vi "geve-init.vi"(8 "error in (no error)":errorcluster) -> (0 "error out":errorcluster, 3 "Runtime Data":T1)   [LabVIEW 2018]
doc: "perfoms action :\ninit com references,\nenqueue message append init message to log\nget configuration from cfg file, enqueue message to log info and to update data in main cluster\nenqueue message to open serial com."
uses:
  geve-runtime_data_cluster.ctl
  geve-monitoring_data_cluster.ctl
  geve-serial_config_cluster.ctl
  geve-com_ref_cluster.ctl
  geve-message_cluster.ctl
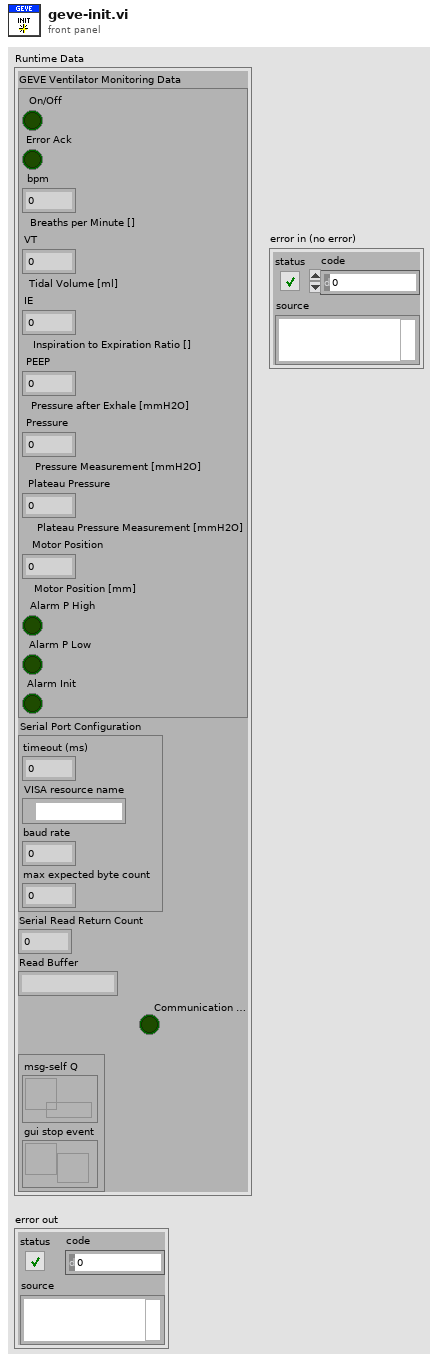
[diagram p1: front panel]
types:
  T1 = typedef "geve-runtime_data_cluster.ctl" = cluster{"GEVE Ventilator Monitoring Data":T2, "Serial Port Configuration":T3, "Serial Read Return Count":u32, "Read Buffer":string, "Communication Timeout?":bool, "com-refs":T4}
  T2 = typedef "geve-monitoring_data_cluster.ctl" = cluster{"On/Off":bool, "Error Ack":bool, "bpm":dbl, "VT":dbl, "IE":dbl, "PEEP":dbl, "Pressure":dbl, "Plateau Pressure":dbl, "Motor Position":dbl, "Alarm P High":bool, "Alarm P Low":bool, "Alarm Init":bool}
  T3 = typedef "geve-serial_config_cluster.ctl" = cluster{"timeout (ms)":u32, "VISA resource name":refnum<visa-resource-name>, "baud rate":u32, "max expected byte count":u32}
  T4 = typedef "geve-com_ref_cluster.ctl" = cluster{"msg-self Q":refnum<queue>, "gui stop event":refnum<user-event>}
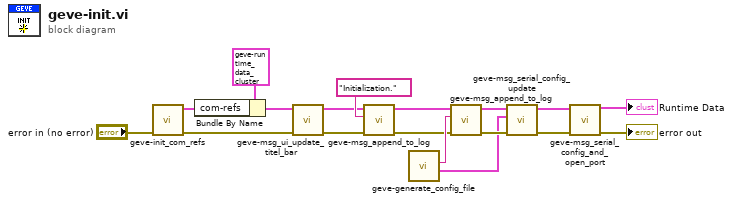
[diagram p0: block diagram]
diagram:
  n1 = call "geve-init_com_refs.vi"("error in (no error)"="error in (no error)") -> ("error out"=w10:errorcluster, "com-refs"=w8:T4)  [unwired: 9 in]
  n2 = Bundle By Name(cluster=T1 {"GEVE Ventilator Monitoring Data"={"On/Off"=FALSE, "Error Ack"=FALSE, "bpm"=0.0, "VT"=0.0, "IE"=0.0, "PEEP"=0.0, "Pressure"=0.0, "Plateau Pressure"=0.0, "Motor Position"=0.0, "Alarm P High"=FALSE, "Alarm P Low"=FALSE, "Alarm Init"=FALSE}, "Serial Port Configuration"={"timeout (ms)"=0, "VISA resource name"="", "baud rate"=0, "max expected byte count"=128}, "Serial Read Return Count"=0, "Read Buffer"="", "Communication Timeout?"=FALSE, "com-refs"={"msg-self Q"=refnum, "gui stop event"=refnum}} ("Runtime Data"), "com-refs"=w8) -> (w7:T1)
  n3 = call "geve-msg_ui_update_titel_bar.vi"("error in (no error)"=w10, "Runtime Data"=w7) -> ("error out"=w17:errorcluster, "Runtime Data out"=w13:T1)  [unwired: 8 in]
  n4 = call "geve-msg_append_to_log.vi"("error in (no error)"=w17, "Status Message"="Initialization.", "Runtime Data"=w13) -> ("error out"=w1:errorcluster, "Runtime Dataout"=w2:T1)  [unwired: 7 in]
  n5 = call "geve-generate_config_file.vi"() -> ("serial cfg"=w4:T3, "info"=w6:string)  [unwired: 9 in, 1 out]
  n6 = call "geve-msg_append_to_log.vi"("error in (no error)"=w1, "Status Message"=w6, "Runtime Data"=w2) -> ("error out"=w5:errorcluster, "Runtime Dataout"=w3:T1)  [unwired: 7 in]
  n7 = call "geve-msg_serial_config_update.vi"("error in (no error)"=w5, "Serial Port Configuration"=w4, "Runtime Data"=w3) -> ("error out"=w18:errorcluster, "Runtime Data out"=w12:T1)  [unwired: 7 in]
  n8 = call "geve-msg_serial_config_and_open_port.vi"("error in (no error)"=w18, "Runtime Data"=w12) -> ("error out"=→"error out":errorcluster, "Runtime Data out"=→"Runtime Data":T1)  [unwired: 8 in]
